vi "中英切换（菜单+控件标签）.vi"() -> ()   [LabVIEW 2016]
panel:
  in  "字符串":string caption="zifuchuang"
  out "指示灯":bool caption="zhishideng"
  in  "运行时菜单路径(中文)":path caption="母鸡啊2"
  in  "停止":bool caption="母鸡啊3"
  in  "运行时菜单路径（英文）":path caption="母鸡啊"
  in  "语言切换":bool caption="母鸡啊4"
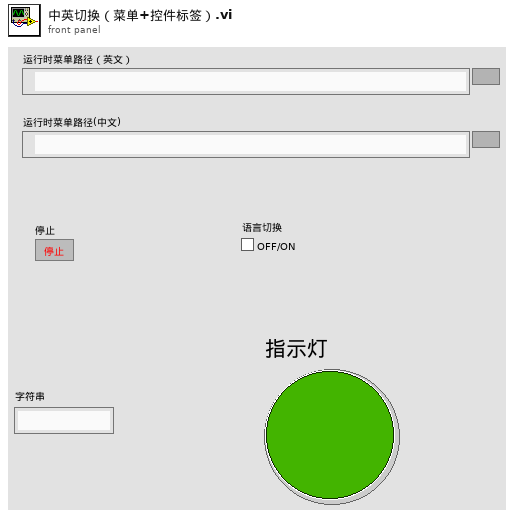
[diagram p1: front panel]
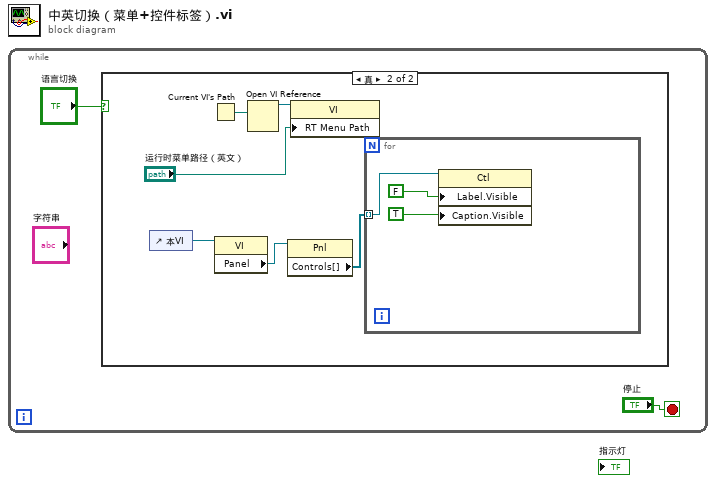
[diagram p0: block diagram]
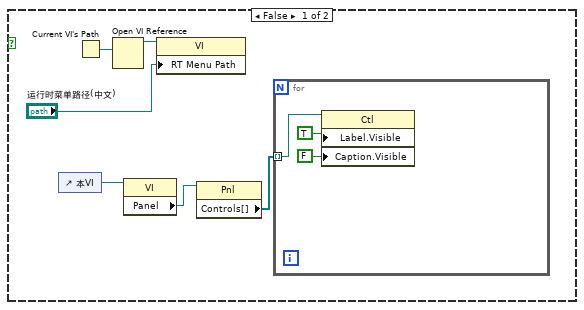
[diagram p2: hidden frame]
diagram:
  n1 = while {
    stop <- "停止" stop-if-true
    n2 = case shown="真" "语言切换" {
      frame False {
        n3 = control-ref of="本VI"() -> (w5:refnum<vi>)
        n4 = Current VI's Path() -> (path=w7:path)
        n5 = Open VI Reference(vi path=w7) -> (vi reference=w8:refnum<vi>)  [unwired: 5 in, 1 out]
        n6 = property class="VI"(reference=w5) -> ("Panel"=w4:refnum<vi>)  [unwired: 1 in, 2 out]
        n7 = property class="VI"(reference=w8, "RT Menu Path"="运行时菜单路径(中文)") -> ()  [unwired: 1 in, 2 out]
        n8 = property class="Pnl"(reference=w4) -> ("Controls[]"=w3:refnum<vi>[])  [unwired: 1 in, 2 out]
        n9 = for {
          tunnel: w3 -> [w11] mode=indexing
          n10 = property class="Ctl"(reference=w11, "Label.Visible"=TRUE ("标签.可见"), "Caption.Visible"=FALSE ("标题.可见")) -> ()  [unwired: 1 in, 2 out]
        }
      }
      frame True {
        n11 = control-ref of="本VI"() -> (w14:refnum<vi>)
        n12 = Current VI's Path() -> (path=w16:path)
        n13 = property class="VI"(reference=w14) -> ("Panel"=w13:refnum<vi>)  [unwired: 1 in, 2 out]
        n14 = Open VI Reference(vi path=w16) -> (vi reference=w17:refnum<vi>)  [unwired: 5 in, 1 out]
        n15 = property class="Pnl"(reference=w13) -> ("Controls[]"=w12:refnum<vi>[])  [unwired: 1 in, 2 out]
        n16 = property class="VI"(reference=w17, "RT Menu Path"="运行时菜单路径（英文）") -> ()  [unwired: 1 in, 2 out]
        n17 = for {
          tunnel: w12 -> [w20] mode=indexing
          n18 = property class="Ctl"(reference=w20, "Label.Visible"=FALSE ("标签.可见"), "Caption.Visible"=TRUE ("标题.可见")) -> ()  [unwired: 1 in, 2 out]
        }
      }
    }
  }
